vi "Configure Filters.vi"(7 "Name Filters":string[](array[string]), 8 "error in (no error)":errorcluster, 11 "CD Build Tools in":refnum<class "Project Build Tools.lvclass">) -> (0 "error out":errorcluster, 3 "CD Build Tools out":refnum<class "Project Build Tools.lvclass">)   [LabVIEW 2019, in "Project Build Tools.lvclass"]
uses:
  Project Build Tools.lvclass
  Project Build Tools.lvclass/Project Build Tools.ctl
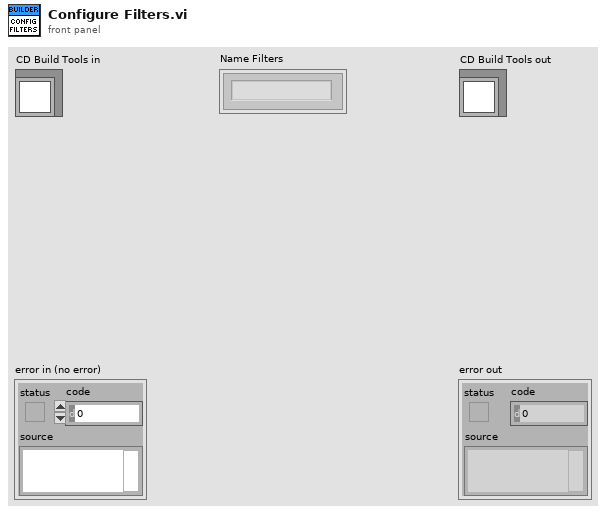
[diagram p1: front panel]
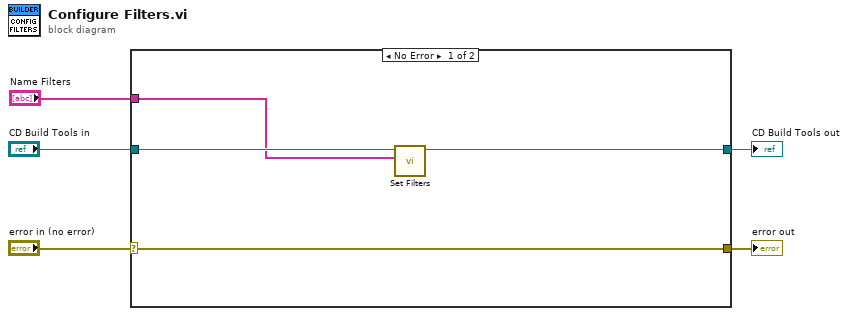
[diagram p0: block diagram]
diagram:
  n1 = case shown="No Error" "error in (no error)" {
    selector: "error in (no error)" -> [w9 w11]
    tunnel: [w9 w11] -> w4
    tunnel: [w6 w10] -> w2
    tunnel: "CD Build Tools in" -> [w8 w10]
    tunnel: "Name Filters" -> [w7 _]
    frame No Error {
      n2 = call "Set Filters.vi"("Filters"=w7, "CD Build Tools in"=w8) -> ("CD Build Tools out"=w6:refnum<class "Project Build Tools.lvclass">)  [unwired: 9 in]
    }
    frame Error {
    }
  }
  "error out" <- w4
  "CD Build Tools out" <- w2
